vi "CRYGet Real CurveName.vi"(9 "Key No":i32, 10 "Additive Info":T2, 11 "CurveArrayByType":string[](array[string])) -> (3 "Curve Info Array Out":T1)   [LabVIEW 2013]
uses:
  Typedef Control/CRYAnalysis CurveName Cluster.ctl
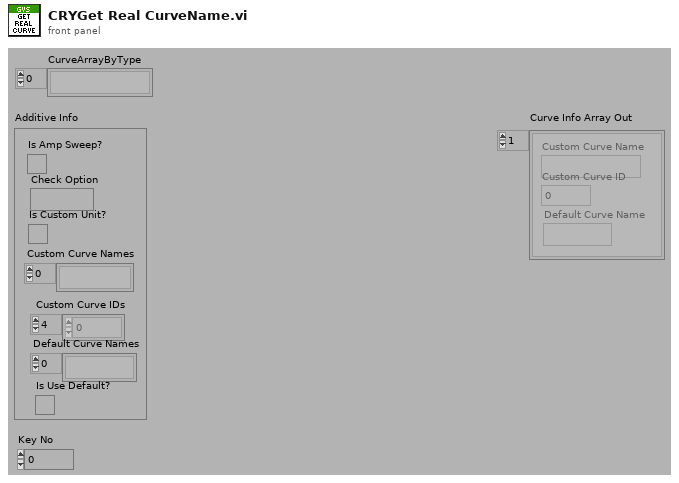
[diagram p1: front panel]
types:
  T1 = typedef "CRYAnalysis CurveName Cluster.ctl" = cluster{"Custom Curve Name":string, "Custom Curve ID":i32, "Default Curve Name":string}[]
  T2 = cluster{"Is Amp Sweep?":bool, "Check Option":string, "Is Custom Unit?":bool, "Custom Curve Names":string[], "Custom Curve IDs":i32[], "Default Curve Names":string[], "Is Use Default?":bool}
  T3 = cluster{"Custom Curve Names":string, "Custom Curve IDs":i32, "Default Curve Names":string}
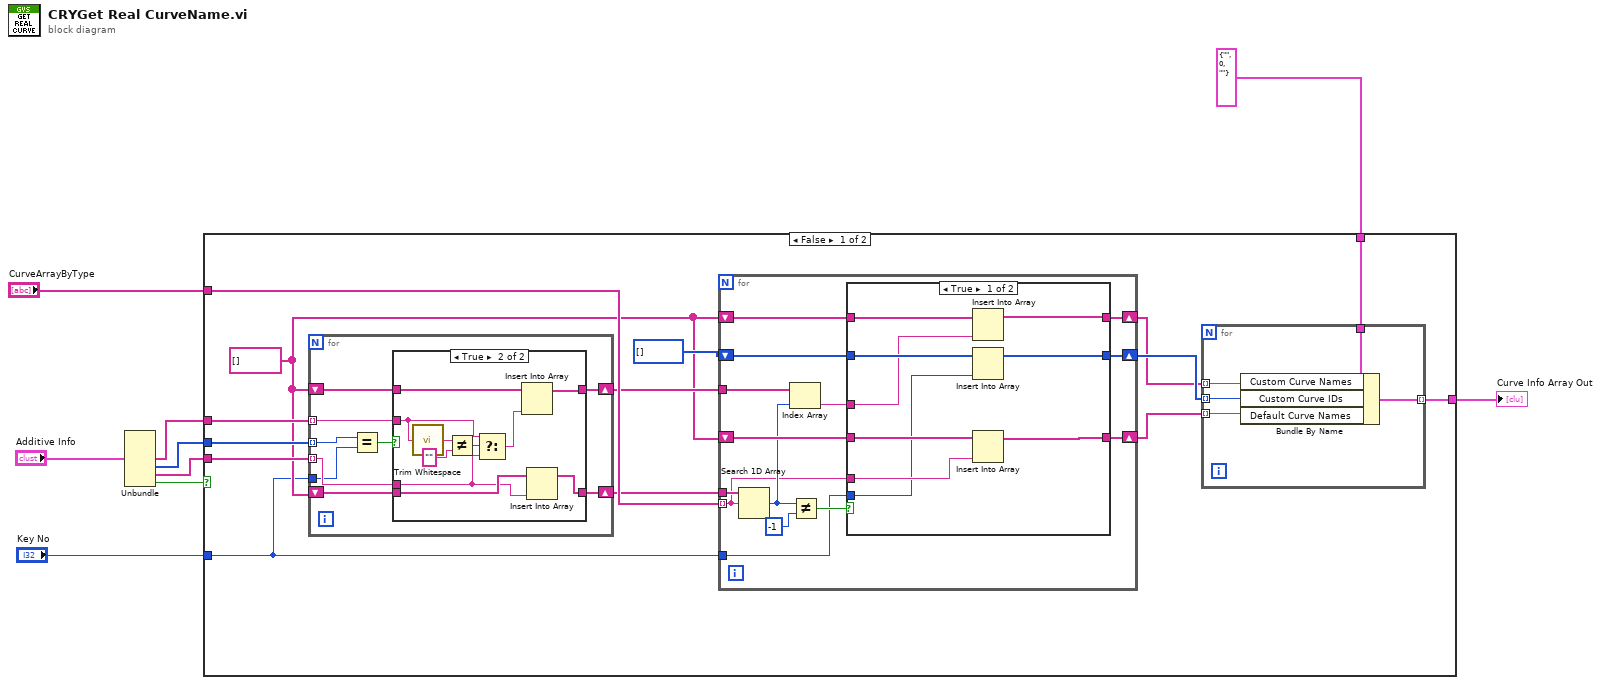
[diagram p0: block diagram]
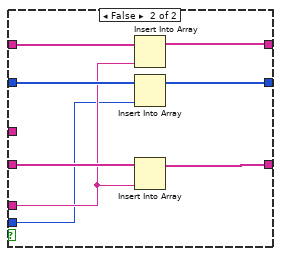
[diagram p3: hidden frame]
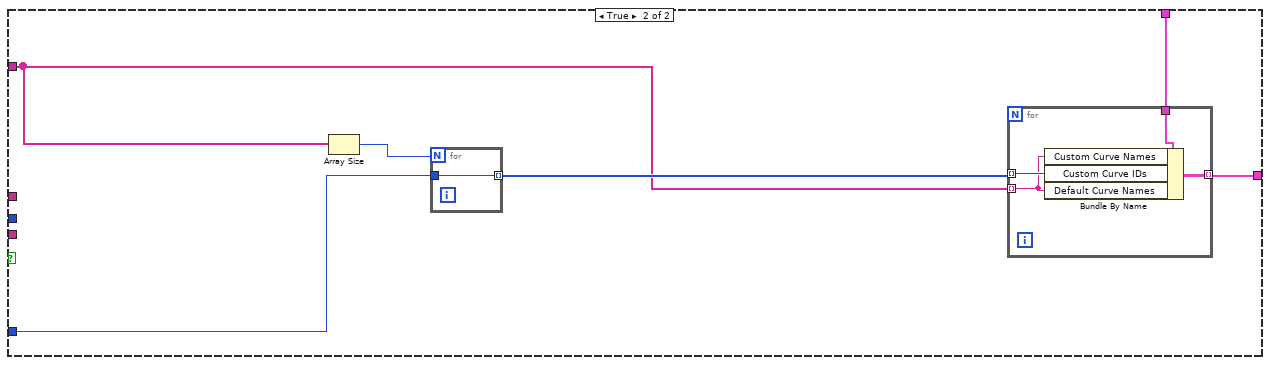
[diagram p4: hidden frame]
diagram:
  n1 = Unbundle("Additive Info") -> ("Custom Curve Names"=w5:string[], "Custom Curve IDs"=w6:i32[], "Default Curve Names"=w7:string[], "Is Use Default?"=w8:bool)  [unwired: 3 out]
  n2 = case shown="False" w8 {
    tunnel: "CurveArrayByType" -> [w23 w82]
    tunnel: w7 -> [w21 _]
    tunnel: w6 -> [w22 _]
    tunnel: w5 -> [w20 _]
    tunnel: [w13 w84] -> w1
    tunnel: "Key No" -> [w12 w83]
    tunnel: T3 {"Custom Curve Names"="", "Custom Curve IDs"=0, "Default Curve Names"=""} ("Cluster") -> [w10 w81]
    frame False {
      w16 = string[] [] ("Custom Curve Names")
      n3 = for {
        tunnel: w22 -> [w30] mode=indexing
        tunnel: w21 -> [w36] mode=indexing
        tunnel: w20 -> [w37] mode=indexing
        shift-right: [w33] -> w19
        shift-left: w16 -> [w34]
        shift-right: [w32] -> w18
        shift-left: w16 -> [w35]
        tunnel: w12 -> [w29]
        n4 = Equal?(x=w30, y=w29) -> (x = y?=w31:bool)
        n5 = case shown="True" w31 {
          tunnel: w37 -> [_ w42]
          tunnel: w36 -> [_ w41]
          tunnel: w35 -> [w38 w47]
          tunnel: w34 -> [w39 w49]
          tunnel: [w39 w48] -> w33
          tunnel: [w38 w46] -> w32
          frame False {
          }
          frame True {
            n6 = call <vilib>:"Trim Whitespace.vi"("string"=w42) -> ("trimmed string"=w45:string)  [unwired: 1 in]
            n7 = Not Equal?(x=w45, y="") -> (x != y?=w43:bool)
            n8 = Select(t=w42, s=w43, f=w41) -> (s? t:f=w40:string)
            n9 = Insert Into Array(array=w49, new element=w40) -> (w48:string[])  [unwired: 1 in]
            n10 = Insert Into Array(array=w47, new element=w41) -> (w46:string[])  [unwired: 1 in]
          }
        }
      }
      n11 = for {
        tunnel: w23 -> [w51] mode=indexing
        tunnel: w19 -> [w54]
        tunnel: w18 -> [w63]
        shift-right: [w57] -> w11
        shift-left: w16 -> [w60]
        shift-right: [w56] -> w15
        shift-left: i32[] [] ("Custom Curve IDs") -> [w59]
        shift-right: [w55] -> w14
        shift-left: w16 -> [w58]
        tunnel: w12 -> [w50]
        n12 = Search 1D Array(1D array=w63, element=w51) -> (index of element=w53:i32)  [unwired: 1 in]
        n13 = Index Array(array=w54, index=w53) -> (element=w52:string)
        n14 = Not Equal?(x=w53, y=-1) -> (x != y?=w61:bool)
        n15 = case shown="True" w61 {
          tunnel: w60 -> [w67 w76]
          tunnel: w59 -> [w69 w78]
          tunnel: w58 -> [w72 w80]
          tunnel: [w66 w75] -> w57
          tunnel: [w68 w77] -> w56
          tunnel: [w71 w79] -> w55
          tunnel: w52 -> [w65 _]
          tunnel: w51 -> [w70 w74]
          tunnel: w50 -> [w64 w73]
          frame True {
            n16 = Insert Into Array(array=w67, new element=w65) -> (w66:string[])  [unwired: 1 in]
            n17 = Insert Into Array(array=w69, new element=w64) -> (w68:i32[])  [unwired: 1 in]
            n18 = Insert Into Array(array=w72, new element=w70) -> (w71:string[])  [unwired: 1 in]
          }
          frame False {
            n19 = Insert Into Array(array=w76, new element=w74) -> (w75:string[])  [unwired: 1 in]
            n20 = Insert Into Array(array=w78, new element=w73) -> (w77:i32[])  [unwired: 1 in]
            n21 = Insert Into Array(array=w80, new element=w74) -> (w79:string[])  [unwired: 1 in]
          }
        }
      }
      n22 = for {
        tunnel: w15 -> [w28] mode=indexing
        tunnel: w14 -> [w27] mode=indexing
        tunnel: [w26] -> w13 mode=indexing
        tunnel: w11 -> [w25] mode=indexing
        tunnel: w10 -> [w24]
        n23 = Bundle By Name(cluster=w24, "Custom Curve Names"=w25, "Custom Curve IDs"=w28, "Default Curve Names"=w27) -> (w26:T3)
      }
    }
    frame True {
      n24 = Array Size(array=w82) -> (size(s)=w86:i32)
      n25 = for {
        N: w86 -> [_]
        tunnel: [w91] -> w85 mode=indexing
        tunnel: w83 -> [w91]
      }
      n26 = for {
        tunnel: w85 -> [w90] mode=indexing
        tunnel: [w89] -> w84 mode=indexing
        tunnel: w82 -> [w88] mode=indexing
        tunnel: w81 -> [w87]
        n27 = Bundle By Name(cluster=w87, "Custom Curve Names"=w88, "Custom Curve IDs"=w90, "Default Curve Names"=w88) -> (w89:T3)
      }
    }
  }
  "Curve Info Array Out" <- w1
